vi "Add-log-message-motor.vi"(8 "error in (no error)":errorcluster, 9 "Motor index":i32, 10 "Message":string, 11 "UI in":T1) -> (0 "error out":errorcluster, 3 "UI out":T1)   [LabVIEW 2013, in "PowderDeposition.lvlib" / "PD-Main.lvclass"]
uses:
  PD-Main.lvclass
  Object-reference.ctl
  PD-Main.lvclass/PD-Main.ctl
  Read Activity log.vi
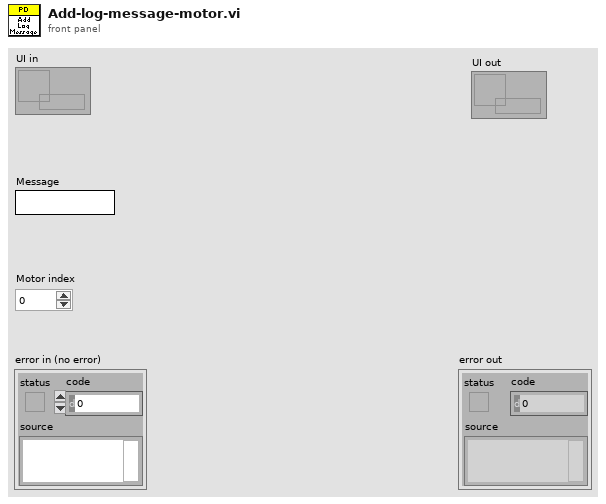
[diagram p1: front panel]
types:
  T1 = typedef "PowderDeposition.lvlib/PD-Main.lvclass/Object-reference.ctl" = refnum<data-value>
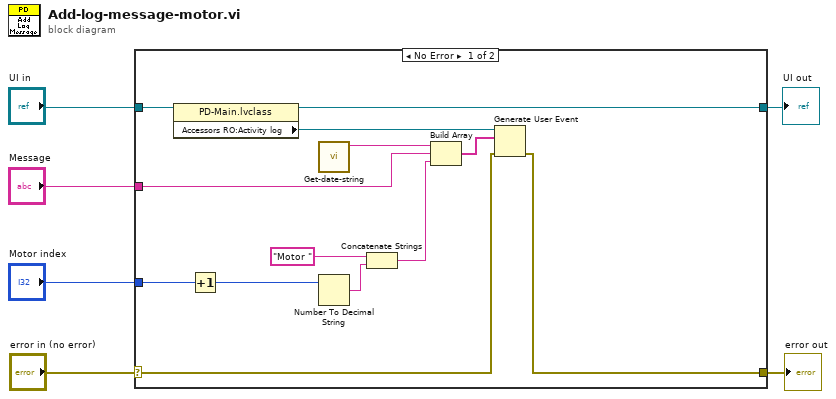
[diagram p0: block diagram]
diagram:
  n1 = case shown="No Error" "error in (no error)" {
    selector: "error in (no error)" -> [w11 w21]
    tunnel: [w10 w21] -> w5
    tunnel: [w9 w20] -> w2
    tunnel: "UI in" -> [w13 w20]
    tunnel: "Message" -> [w18 _]
    tunnel: "Motor index" -> [w17 _]
    frame No Error {
      n2 = property class="PD-Main.lvclass"(reference=w13) -> (reference out=w9:T1, "Accessors RO:Activity log"=w8:refnum<user-event>)  [unwired: 1 in, 1 out]
      n3 = Increment(x=w17) -> (x+1=w7:i32)
      n4 = call "Get-date-string.vi"() -> ("Date string"=w19:string)  [unwired: 11 in]
      n5 = Number To Decimal String(number=w7) -> (decimal integer string=w16:string)  [unwired: 1 in]
      n6 = Concatenate Strings("Motor ", w16) -> (w14:string)
      n7 = Build Array(w19, w18, w14) -> (w12:string[])
      n8 = Generate User Event(user event=w8, event data cluster=w12, error in=w11) -> (error out=w10:errorcluster)  [unwired: 1 in, 1 out]
    }
    frame Error {
    }
  }
  "error out" <- w5
  "UI out" <- w2
